vi "Parse EscapedVariable.vi"(8 "Error In":errorcluster) -> (0 "Error Out":errorcluster)   [LabVIEW 2017, in "Tests.lvlib" / "Parser.lvlib"]
uses:
  Parser.lvlib
  src/Mustache/Public/Tokens/Public/EscapedVariable/EscapedVariable.lvclass
  src/Mustache/Public/Tokens/Public/EscapedVariable/EscapedVariable.lvclass/EscapedVariable.ctl
  src/Mustache/Public/Readers/Public/String/String.lvclass
  D:/Users/cfield/Code/Field R&D Services/Mustache/feature-lv-original-parser/src/Mustache/Public/Readers/Public/Abstract/Abstract.lvclass
  <vilib>/addons/_JKI Toolkits/Caraya/classes/Test/Test.lvclass
  src/Mustache/Public/Parser/Parser.lvclass
  <vilib>/addons/_JKI Toolkits/Caraya/classes/Assert/Assert.lvclass
  src/Mustache/Public/Tokens/Public/Abstract/Abstract.lvclass
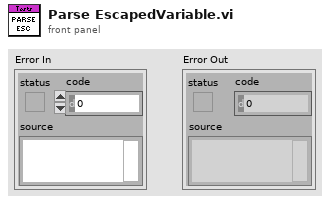
[diagram p1: front panel]
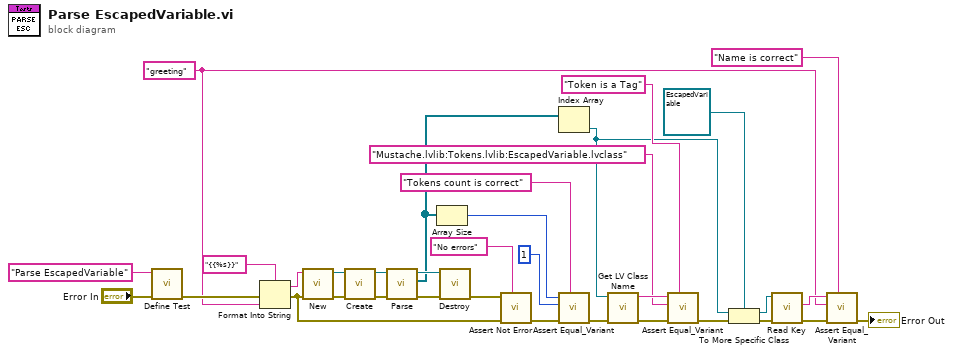
[diagram p0: block diagram]
diagram:
  w3 = "greeting"
  n1 = call <vilib>:"Define Test.vi"("error in (no error)"="Error In", "Label (VI Title)"="Parse EscapedVariable") -> ("error out"=w25:errorcluster)  [unwired: 9 in]
  n2 = Format Into String(format string="{{%s}}", error in=w25, w3) -> (resulting string=w1:string, error out=w4:errorcluster)  [unwired: 1 in]
  n3 = call "New.vi"("Error In"=w4, "String"=w1) -> ("Error Out"=w31:errorcluster, "String"=w32:refnum<class "String.lvclass">)  [unwired: 8 in]
  n4 = call "Create.vi"("Error In"=w31, "Reader"=w32) -> ("Error Out"=w30:errorcluster, "Parser"=w29:refnum<class "Parser.lvclass">)  [unwired: 8 in]
  n5 = call "Parse.vi"("Error In"=w30, "Parser In"=w29) -> ("Error Out"=w27:errorcluster, "Tokens"=w19:refnum<class "Abstract.lvclass">[], "Parser Out"=w28:refnum<class "Parser.lvclass">)  [unwired: 7 in]
  n6 = Array Size(array=w19) -> (size(s)=w21:i32)
  n7 = call "Destroy.vi"("Error In"=w27, "Parser"=w28) -> ("Error Out"=w26:errorcluster)  [unwired: 9 in]
  n8 = call <vilib>:"Assert Not Error.vi"("Label"="No errors", "error in (no error)"=w4, "Not Error?"=w26) -> ("error out"=w23:errorcluster)  [unwired: 8 in]
  n9 = Index Array(array=w19) -> (element=w12:refnum<class "Abstract.lvclass">)  [unwired: 1 in]
  n10 = call <vilib>:"Assert Equal_Variant.vi"("Label"="Tokens count is correct", "error in (no error)"=w23, "Y"=1 ("size(s)"), "X"=w21) -> ("error out"=w17:errorcluster)  [unwired: 7 in]
  n11 = call <vilib>:"Get LV Class Name.vi"("error in (no error)"=w17, "object"=w12) -> ("error out"=w16:errorcluster, "class name"=w15:string)  [unwired: 8 in]
  n12 = call <vilib>:"Assert Equal_Variant.vi"("Label"="Token is a Tag", "error in (no error)"=w16, "Y"="Mustache.lvlib:Tokens.lvlib:EscapedVariable.lvclass", "X"=w15) -> ("error out"=w13:errorcluster)  [unwired: 7 in]
  n13 = To More Specific Class(target class=refnum<class "EscapedVariable.lvclass"> refnum ("Mustache.lvlib:Tokens.lvlib:Tag.lvclass"), reference=w12, error in=w13) -> (specific class reference=w9:refnum<class "EscapedVariable.lvclass">, error out=w10:errorcluster)
  n14 = call "Read Key.vi"("Error In"=w10, "Tag In"=w9) -> ("Error Out"=w6:errorcluster, "Key"=w7:string)  [unwired: 7 in, 1 out]
  n15 = call <vilib>:"Assert Equal_Variant.vi"("Label"="Name is correct", "error in (no error)"=w6, "Y"=w3, "X"=w7) -> ("error out"=→"Error Out":errorcluster)  [unwired: 7 in]
